vi "Backup.vi"() -> ()   [LabVIEW 2019]
uses:
  D2XX_HeaterStage/D2XX_HeaterStage.lvlib
  <userlib>/LevyLab/Relay Box/D2XX_Functions/D2XX_Functions.lvlib
panel:
  in  "Numeric":i32
  out "error out":errorcluster
  in  "error in (no error)":errorcluster
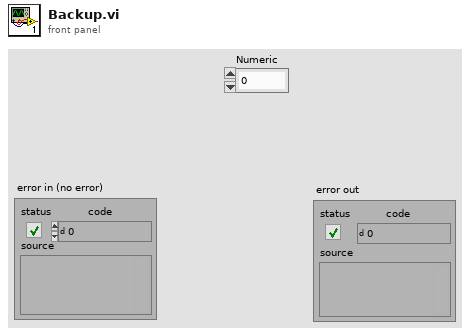
[diagram p1: front panel]
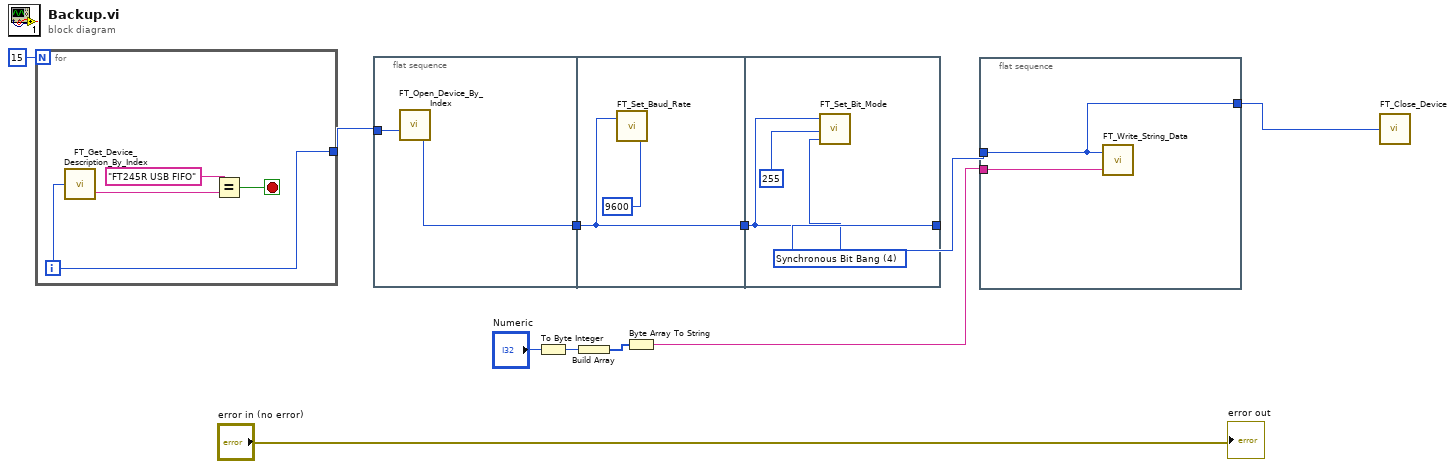
[diagram p0: block diagram]
diagram:
  n1 = for {
    N: 15 -> [_]
    tunnel: [w12] -> w7
    i -> [w12]
    stop <- w13 stop-if-true
    n2 = call "FT_Get_Device_Description_By_Index.vi"("Device Index"=w12) -> ("Device Description"=w14:string)  [unwired: 1 out]
    n3 = Equal?(x="FT245R USB FIFO", y=w14) -> (x = y?=w13:bool)
  }
  n4 = flat-sequence {
    tunnel: w7 -> [w17]
    tunnel: [w16] -> w11
    tunnel: w11 -> [w19]
    tunnel: [w19] -> w10
    tunnel: [w22] -> w3
    tunnel: w10 -> [w22]
    frame #0 {
      n5 = call "FT_Open_Device_By_Index.vi"("Device Index"=w17) -> ("Handle"=w16:u32)  [unwired: 1 out]
    }
    frame #1 {
      n6 = call <userlib>:"FT_Set_Baud_Rate.vi"("Baud Rate"=u32 9600, "Handle"=w19) -> ()  [unwired: 1 out]
    }
    frame #2 {
      w20 = u8 4 items=["Reset Bit Mode"=0, "Asynchronous Bit Bang"=1, "MPSSE"=2, "Synchronous Bit Bang"=4, "MCU Host Bus Emulation"=8, "Fast Opto-Isolated Serial"=16, "CBUS Bit Bang"=32, "Single Channel 245 Synchronous FIFO"=64] ("Bit Mode")
      n7 = call <userlib>:"FT_Set_Bit_Mode.vi"("Bit Mode"=w20, "Bit Mode Mask"=u8 255, "Handle"=w22) -> ()  [unwired: 1 out]
    }
  }
  n8 = To Byte Integer(number="Numeric") -> (8bit integer=w6:i8)
  n9 = Build Array(w6) -> (w5:i8[])
  n10 = Byte Array To String(unsigned byte array=w5) -> (string=w4:string)
  n11 = flat-sequence {
    tunnel: w3 -> [w24]
    tunnel: [w24] -> w8
    tunnel: w4 -> [w23]
    frame #0 {
      n12 = call "FT_Write_String_Data.vi"("Buffer"=w23, "Handle"=w24) -> ()  [unwired: 2 out]
    }
  }
  n13 = call "FT_Close_Device.vi"("Handle"=w8) -> ()  [unwired: 1 out]
  "error out" <- "error in (no error)"
